vi "Serial Port Open.vi"(8 "error in (no error)":errorcluster, 11 "Port name (COM1)":string="COM1") -> (0 "error out":errorcluster, 3 "Port handle":refnum<k24>)   [LabVIEW 2015, in "VC940.lvlib"]
uses:
  VC940.lvlib
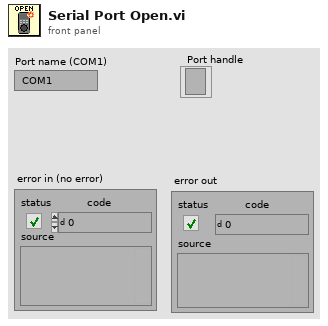
[diagram p1: front panel]
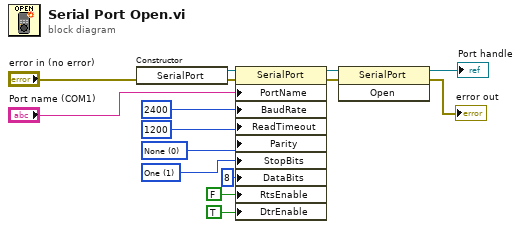
[diagram p0: block diagram]
diagram:
  w12 = 1 items=["None", "One", "Two", "OnePointFive"] ("StopBits")
  w11 = 0 items=["None", "Odd", "Even", "Mark", "Space"] ("Parity")
  n1 = constructor class="SerialPort"(error in="error in (no error)") -> (reference out=w5:refnum<k24>, error out=w4:errorcluster)  [unwired: 2 in, 1 out]
  n2 = property class="SerialPort"(reference=w5, error in=w4, "PortName"="Port name (COM1)", "BaudRate"=2400, "ReadTimeout"=1200, "Parity"=w11, "StopBits"=w12, "DataBits"=8, "RtsEnable"=FALSE, "DtrEnable"=TRUE ("RtsEnable")) -> (reference out=w8:refnum<k24>, error out=w7:errorcluster)
  n3 = invoke class="SerialPort" method="Open"(reference=w8, error in=w7) -> (reference out=→"Port handle":refnum<k24>, error out=→"error out":errorcluster)  [unwired: 1 in, 1 out]
